vi "AIT 664 - Parse Tree Messages.vi"(0 "Device Reference in":T7 format="%.0x", 2 "Access Type":T8=enum."Write", 5 "Message Reference in":T7 format="%.0x", 7 "FIFO Index Queues in":T9, 11 "error in":errorcluster) -> (4 "Message Settings out":T1={"Name"="", "xmlName"="", "Tx-Rx_T-Tx"=FALSE, "RT_Address"=0, "RT_SA_Address"=0, "Block Data Refs"=[], "Values Array"=[], "Length"=0, "Words"=0, "FIFO Index"=0, "RX Word"=0, "IterationOffset"=0, "Default Msg Data"=[], "Driver Data"={"First Word"=[], "Start Bit"=[], "Num Bits"=[], "Decimation"=0, "IterationOffset"=0, "Signed?"=[], "ScaleFac"=[], "ScaleOffset"=[]}, "Status Data"=[], "Queue Transmit Channel"=18446744073709551615, "Transmit Channel Data Reference"=0} {"Transmit Channel Data Reference" format="%.0x"; "Queue Transmit Channel" format="%.0x"; "Driver Data"."Num Bits" min=1 max=32; "Block Data Refs"."Data Reference" format="%.0x"}, 6 "Message Name out":string, 15 "error out":errorcluster)   [LabVIEW 2013, in "AIT 664 Custom Device.lvlib"]
doc: "For a given port build up all of the channels, which include user defined channels and status information."
uses:
  AIT 664 Custom Device.lvlib
  <vilib>/NI Veristand/Custom Device API/Custom Device Item Ref.ctl
  RT Controls/FIFO Index Queues.ctl
  <vilib>/NI Veristand/Custom Device API/Data Access Type.ctl
  RT Controls/AIT 664 - RT Message Settings.ctl
  <vilib>/NI Veristand/Custom Device API/Block Data Reference.ctl
  <vilib>/NI Veristand/Custom Device API/Data Reference.ctl
  RT Controls/AIT 664 - Driver Data.ctl
  Controls and Global/Start Bit.ctl
  Controls and Global/Number of Bits.ctl
  RT Controls/Data Ref FGV Command.ctl
  <vilib>/NI Veristand/Custom Device Tools/Custom Device Utility Library/NI VeriStand - Search for Item.vi
  <vilib>/NI Veristand/Custom Device Tools/Custom Device Utility Library/NI VeriStand - Search for All Items by GUID.vi
  Controls and Global/Global.vi
  <vilib>/NI Veristand/Custom Device API/NI VeriStand - Get Item Property.vi
  <vilib>/NI Veristand/Custom Device API/Get Item Property (Double).vi
  <vilib>/NI Veristand/Custom Device API/Get Item Property (Boolean).vi
  <vilib>/NI Veristand/Custom Device API/Get Item Property (I32).vi
  <vilib>/NI Veristand/Custom Device Tools/Custom Device Utility Library/NI VeriStand - Search for Item by GUID.vi
  <vilib>/NI Veristand/Custom Device API/Custom Device API.lvlib
  <vilib>/NI Veristand/Custom Device Tools/Custom Device Utility Library/Custom Device Utility Library.lvlib
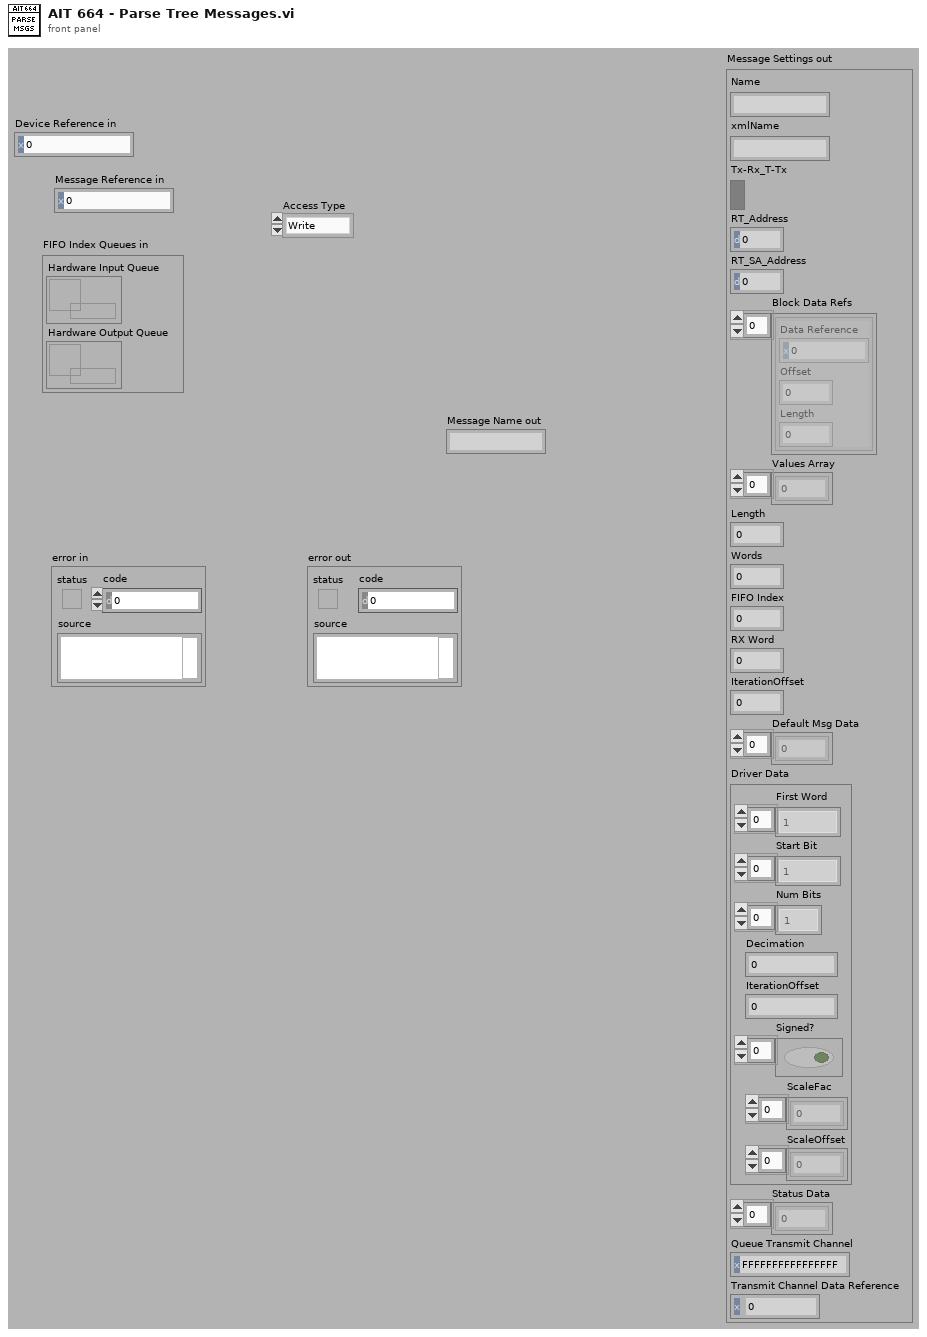
[diagram p1: front panel]
types:
  T1 = typedef "AIT 664 Custom Device.lvlib/AIT 664 - RT Message Settings.ctl" = cluster{"Name":string, "xmlName":string, "Tx-Rx_T-Tx":bool, "RT_Address":u8, "RT_SA_Address":u8, "Block Data Refs":T2[], "Values Array":dbl[], "Length":i32, "Words":i32, "FIFO Index":i32, "RX Word":u32, "IterationOffset":i32, "Default Msg Data":u8[], "Driver Data":T4, "Status Data":u32[], "Queue Transmit Channel":T7, "Transmit Channel Data Reference":T3}
  T2 = typedef "Custom Device API.lvlib/Block Data Reference.ctl" = cluster{"Data Reference":T3, "Offset":i32, "Length":i32}
  T3 = typedef "Custom Device API.lvlib/Data Reference.ctl" = i32
  T4 = typedef "AIT 664 Custom Device.lvlib/AIT 664 - Driver Data.ctl" = cluster{"First Word":T5[], "Start Bit":T5[], "Num Bits":T6[], "Decimation":i32, "IterationOffset":i32, "Signed?":bool[], "ScaleFac":dbl[], "ScaleOffset":dbl[]}
  T5 = typedef "AIT 664 Custom Device.lvlib/Start Bit.ctl" = i32
  T6 = typedef "AIT 664 Custom Device.lvlib/Number of Bits.ctl" = i32
  T7 = typedef "Custom Device API.lvlib/Custom Device Item Ref.ctl" = u64
  T8 = typedef "Custom Device API.lvlib/Data Access Type.ctl" = enum16{"Read", "Write"}
  T9 = typedef "AIT 664 Custom Device.lvlib/FIFO Index Queues.ctl" = cluster{"Hardware Input Queue":refnum<queue>, "Hardware Output Queue":refnum<queue>}
  T10 = typedef "Custom Device API.lvlib/Custom Device Item Info.ctl" = cluster{"Name":string, "Is Channel":bool, "GUID":string, "Is Waveform":bool}
  T11 = typedef "AIT 664 Custom Device.lvlib/Data Ref FGV Command.ctl" = enum16{"Intialize", "Get", "Update"}
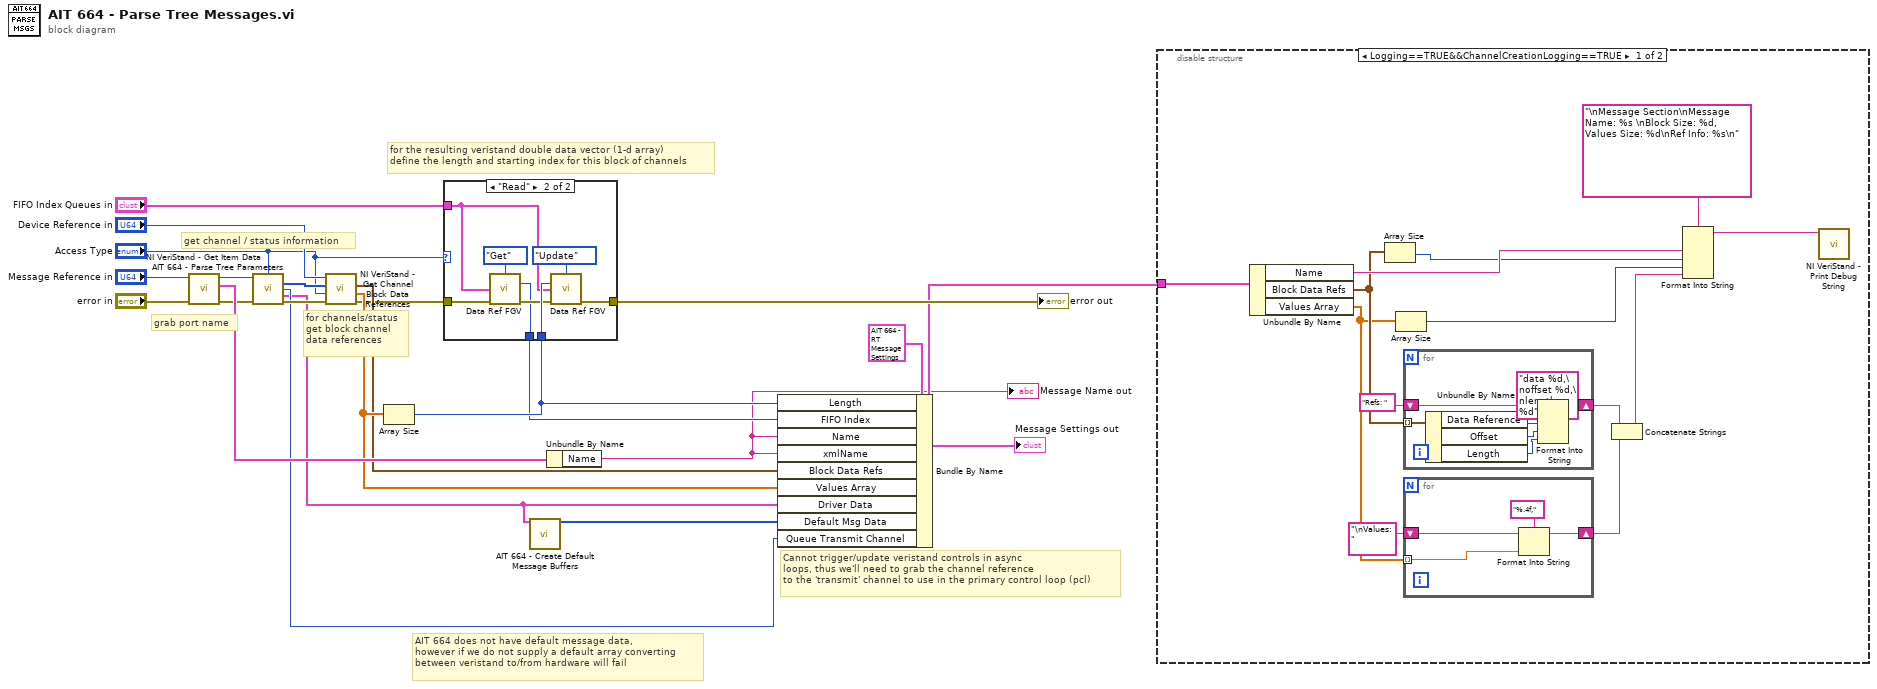
[diagram p0: block diagram]
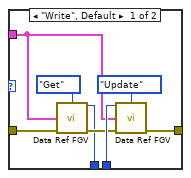
[diagram p2: hidden frame]
diagram:
  # "Cannot trigger/update veristand controls in async\nloops, thus we'll need to grab the channel reference\nto the 'transmit' channel to use in the primary control loop (pcl)"
  # "for the resulting veristand double data vector (1-d array)\ndefine the length and starting index for this block of channels"
  # "for channels/status\nget block channel \ndata references"
  # "get channel / status information"
  # "grab port name"
  # "AIT 664 does not have default message data,\nhowever if we do not supply a default array converting\nbetween veristand to/from hardware will fail"
  n1 = call <vilib>:"NI VeriStand - Get Item Data.vi"("error in (no error)"="error in", "Item Ref in"="Message Reference in") -> ("error out"=w18:errorcluster, "Item Info"=w19:T10, "Item Ref out"=w17:T7)  [unwired: 6 in, 1 out]
  n2 = call "AIT 664 - Parse Tree Parameters.vi"("Item Ref in"=w17, "Access Type"="Access Type", "error in"=w18) -> ("Parameter References out"=w7:T7[], "Queue Transmit Channel out"=w3:T7, "Parameter Driver Data out"=w1:T4, "error out"=w5:errorcluster)  [unwired: 9 in]
  n3 = call <vilib>:"NI VeriStand - Get Channel Block Data References.vi"("error in (no error)"=w5, "Access"="Access Type", "Channel Refs"=w7, "Device Ref in"="Device Reference in") -> ("error out"=w11:errorcluster, "Values Array"=w15:dbl[], "Block Data Refs"=w14:T2[])  [unwired: 4 in, 1 out]
  n4 = Array Size(array=w15) -> (size(s)=w13:i32)
  n5 = case shown="\"Read\"" "Access Type" {
    tunnel: w11 -> [w27 w35]
    tunnel: [w29 w37] -> w21
    tunnel: w13 -> [w28 w36]
    tunnel: "FIFO Index Queues in" -> [w25 w32]
    tunnel: [w23 w33] -> w12
    frame "Write", Default {
      n6 = call "Data Ref FGV.vi"("Action"=Data_Ref_FGV_Command."Get" ("Command"), "FIFO Index Queues"=w25, "error in (no error)"=w27) -> ("Hardware Input FIFO Index"=w23:i32, "error out"=w26:errorcluster)  [unwired: 10 in, 1 out]
      n7 = call "Data Ref FGV.vi"("Hardware Input Length in"=w28, "Action"=Data_Ref_FGV_Command."Update" ("Command"), "FIFO Index Queues"=w25, "error in (no error)"=w26) -> ("error out"=w29:errorcluster)  [unwired: 9 in, 2 out]
    }
    frame "Read" {
      n8 = call "Data Ref FGV.vi"("Action"=Data_Ref_FGV_Command."Get" ("Command"), "FIFO Index Queues"=w32, "error in (no error)"=w35) -> ("Hardware Output FIFO Index"=w33:i32, "error out"=w34:errorcluster)  [unwired: 10 in, 1 out]
      n9 = call "Data Ref FGV.vi"("Action"=Data_Ref_FGV_Command."Update" ("Command"), "Hardware Output Length in"=w36, "FIFO Index Queues"=w32, "error in (no error)"=w34) -> ("error out"=w37:errorcluster)  [unwired: 9 in, 2 out]
    }
  }
  "error out" <- w21
  n10 = call "AIT 664 - Create Default Message Buffers.vi"("Parameter Driver Data in"=w1) -> ("Default Message Data out"=w8:u8[])  [unwired: 14 in]
  n11 = Unbundle By Name(w19) -> ("Name"=w9:string)
  "Message Name out" <- w9
  n12 = Bundle By Name(cluster=T1 {"Name"="", "xmlName"="", "Tx-Rx_T-Tx"=FALSE, "RT_Address"=0, "RT_SA_Address"=0, "Block Data Refs"=[], "Values Array"=[], "Length"=0, "Words"=0, "FIFO Index"=0, "RX Word"=0, "IterationOffset"=0, "Default Msg Data"=[], "Driver Data"={"First Word"=[], "Start Bit"=[], "Num Bits"=[], "Decimation"=0, "IterationOffset"=0, "Signed?"=[], "ScaleFac"=[], "ScaleOffset"=[]}, "Status Data"=[], "Queue Transmit Channel"=0, "Transmit Channel Data Reference"=0} ("Message Settings"), "Length"=w13, "FIFO Index"=w12, "Name"=w9, "xmlName"=w9, "Block Data Refs"=w14, "Values Array"=w15, "Driver Data"=w1, "Default Msg Data"=w8, "Queue Transmit Channel"=w3) -> (w10:T1)
  "Message Settings out" <- w10
  n13 = disable-structure shown="Logging==TRUE&&ChannelCreationLogging==TRUE" {
    disable-tunnel: w10 -> [w51 _]
    frame condition #0 (active) {
      n14 = Unbundle By Name(w51) -> ("Name"=w49:string, "Block Data Refs"=w47:T2[], "Values Array"=w43:dbl[])
      n15 = Array Size(array=w47) -> (size(s)=w46:i32)
      n16 = Array Size(array=w43) -> (size(s)=w45:i32)
      n17 = for {
        tunnel: w47 -> [w62] mode=indexing
        shift-right: [w59] -> w42
        shift-left: "Refs: " ("format string") -> [w60]
        n18 = Unbundle By Name(w62) -> ("Data Reference"=w58:T3, "Offset"=w57:i32, "Length"=w56:i32)
        n19 = Format Into String(format string="data %d,\noffset %d,\nlength %d", initial string=w60, w58, w57, w56) -> (resulting string=w59:string)  [unwired: 1 in, 1 out]
      }
      n20 = for {
        tunnel: w43 -> [w52] mode=indexing
        shift-right: [w53] -> w41
        shift-left: "\nValues: " ("format string") -> [w54]
        n21 = Format Into String(format string="%.4f,", initial string=w54, w52) -> (resulting string=w53:string)  [unwired: 1 in, 1 out]
      }
      n22 = Concatenate Strings(w42, w41) -> (w40:string)
      n23 = Format Into String(format string="\nMessage Section\nMessage Name: %s \nBlock Size: %d, Values Size: %d\nRef Info: %s\n", w49, w46, w45, w40) -> (resulting string=w39:string)  [unwired: 2 in, 1 out]
      n24 = call <vilib>:"NI VeriStand - Print Debug String.vi"("Message"=w39) -> ()  [unwired: 10 in, 1 out]
    }
    frame condition #1 {
    }
  }
